vi "Review Recipe for Overlap.vi"(6 "Waypoints":cluster{"x":dbl, "y":dbl, "th":dbl}[](array[cluster]), 8 "Blends":T1[](array[typedef]), 11 "Min R":dbl) -> (0 "Blends out":T1[](array[typedef]), 2 "Linear Info":T2(array[cluster]), 3 "Length (f)":dbl, 4 "Waypoints out":cluster{"x":dbl, "y":dbl, "th":dbl}[](array[cluster]))   [LabVIEW 2018]
uses:
  BlendType.ctl
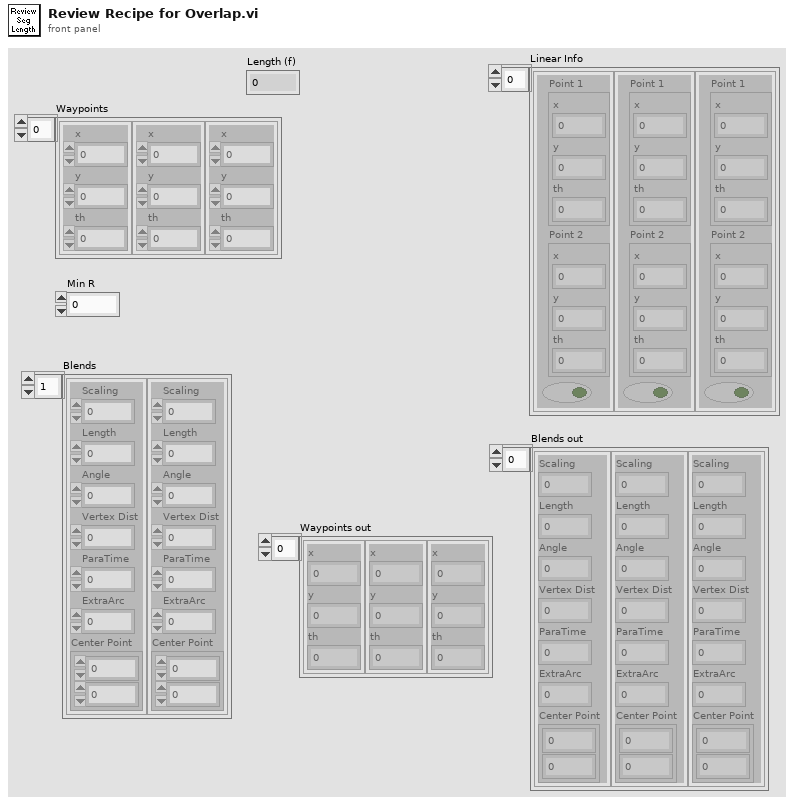
[diagram p1: front panel]
types:
  T1 = typedef "BlendType.ctl" = cluster{"Scaling":dbl, "Length":dbl, "Angle":dbl, "Vertex Dist":dbl, "ParaTime":dbl, "ExtraArc":dbl, "Center Point":cluster{dbl, dbl}}
  T2 = cluster{"Point 1":cluster{"x":dbl, "y":dbl, "th":dbl}, "Point 2":cluster{"x":dbl, "y":dbl, "th":dbl}, bool}[]
  T3 = cluster{"Point Out":cluster{"x":dbl, "y":dbl, "th":dbl}, "Point Out":cluster{"x":dbl, "y":dbl, "th":dbl}, bool}
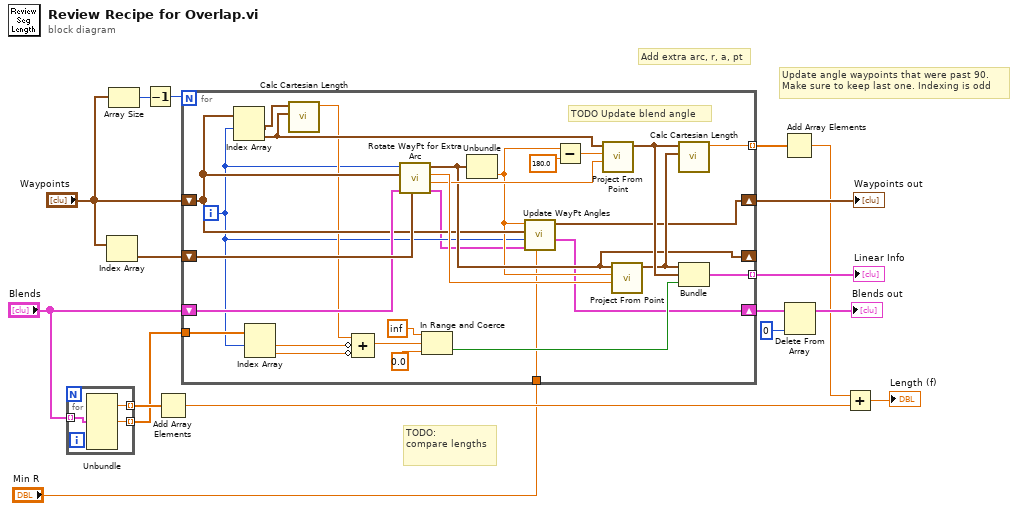
[diagram p0: block diagram]
diagram:
  # "TODO:\ncompare lengths"
  # "Update angle waypoints that were past 90.\nMake sure to keep last one. Indexing is odd"
  # "Add extra arc, r, a, pt"
  n1 = for {
    tunnel: "Blends" -> [w20] mode=indexing
    tunnel: [w19] -> w6 mode=indexing
    tunnel: [w18] -> w5 mode=indexing
    n2 = Unbundle(w20) -> ("Length"=w19:dbl, "Vertex Dist"=w18:dbl)  [unwired: 5 out]
  }
  n3 = Index Array(array="Waypoints") -> (element=w12:cluster{"x":dbl, "y":dbl, "th":dbl})  [unwired: 1 in]
  n4 = Array Size(array="Waypoints") -> (size(s)=w8:i32)
  n5 = Decrement(x=w8) -> (x-1=w9:i32)
  n6 = Add Array Elements(numeric array=w6) -> (sum=w4:dbl)
  n7 = for {
    N: w9 -> [_]
    tunnel: [w48] -> w16 mode=indexing
    tunnel: [w43] -> w17 mode=indexing
    shift-right: [w38] -> _
    shift-left: w12 -> [w42]
    shift-right: [w22] -> w15
    shift-left: "Blends" -> [w41]
    shift-right: [w36] -> w11
    shift-left: "Waypoints" -> [w37]
    tunnel: w5 -> [w34]
    tunnel: "Min R" -> [w21]
    i -> [w24]
    # "TODO Update blend angle"
    n8 = Index Array(array=w37, index #1=w24) -> (element #1=w33:cluster{"x":dbl, "y":dbl, "th":dbl}, element #2=w32:cluster{"x":dbl, "y":dbl, "th":dbl})  [unwired: 1 in]
    n9 = Index Array(array=w34, index #1=w24) -> (element #1=w29:dbl, element #2=w30:dbl)  [unwired: 1 in]
    n10 = call "Calc Cartesian Length.vi"("Point 2"=w32, "Point 1"=w33) -> ("Length (f)"=w31:dbl)  [unwired: 8 in, 1 out]
    n11 = Compound Arithmetic op=ADD(w31, invert w29, invert w30) -> (w28:dbl)
    n12 = call "Rotate WayPt for Extra Arc.vi"("Pt 0"=w42, "Blends In"=w41, "Pts"=w37, "index"=w24) -> ("Blends Out"=w23:T1[], "Pt2 vertex dist"=w39:dbl, "Pt0 vertex dist"=w40:dbl, "Pt Out"=w38:cluster{"x":dbl, "y":dbl, "th":dbl})  [unwired: 4 in]
    n13 = In Range and Coerce(upper limit=inf, x=w28, lower limit=0.0 ("upper limit")) -> (In Range?=w25:bool)  [unwired: 1 out]
    n14 = Unbundle(w38) -> ("th"=w35:dbl)  [unwired: 2 out]
    n15 = call "Update WayPt Angles.vi"("Min R"=w21, "Blends In"=w23, "Index"=w24, "Waypoints in"=w37, "th"=w35) -> ("Blends Out"=w22:T1[], "Waypoints out"=w36:cluster{"x":dbl, "y":dbl, "th":dbl}[])  [unwired: 5 in]
    n16 = Subtract(x=w35, y=180.0) -> (x-y=w47:dbl)
    n17 = call "Project From Point.vi"("distance"=w39, "th"=w47, "Point In"=w32) -> ("Point Out"=w45:cluster{"x":dbl, "y":dbl, "th":dbl})  [unwired: 8 in]
    n18 = call "Project From Point.vi"("distance"=w40, "th"=w35, "Point In"=w38) -> ("Point Out"=w44:cluster{"x":dbl, "y":dbl, "th":dbl})  [unwired: 8 in]
    n19 = call "Calc Cartesian Length.vi"("Point 2"=w44, "Point 1"=w45) -> ("Length (f)"=w43:dbl)  [unwired: 8 in, 1 out]
    n20 = Bundle("Point Out"=w44, "Point Out"=w45, w25) -> (w48:T3)  [unwired: 1 in]
  }
  "Linear Info" <- w16
  "Waypoints out" <- w11
  n21 = Add Array Elements(numeric array=w17) -> (sum=w3:dbl)
  n22 = Delete From Array(array=w15, index=0) -> (array with subset deleted=→"Blends out":T1[])  [unwired: 1 in, 1 out]
  n23 = Add(x=w3, y=w4) -> (x+y=→"Length (f)":dbl)
